vi "load_project.vi"(8 "error in (no error)":errorcluster, 11 "project_file":path) -> (0 "error out":errorcluster, 1 "config":T3, 2 "lv-builder out":refnum<class "lv-builder.lvclass">, 3 "build_spec_info []":T1[](array[typedef]))   [LabVIEW 2015, in "lv-build-interface.lvlib"]
uses:
  lv-build-interface.lvlib
  lv-builder/lv-builder.lvclass
  lv-build/public/_controls/configuration.ctl
  lv-build/public/_controls/build_specification.ctl
  lv-build/public/_controls/build_type.ctl
  lv-build/lv-build.lvlib
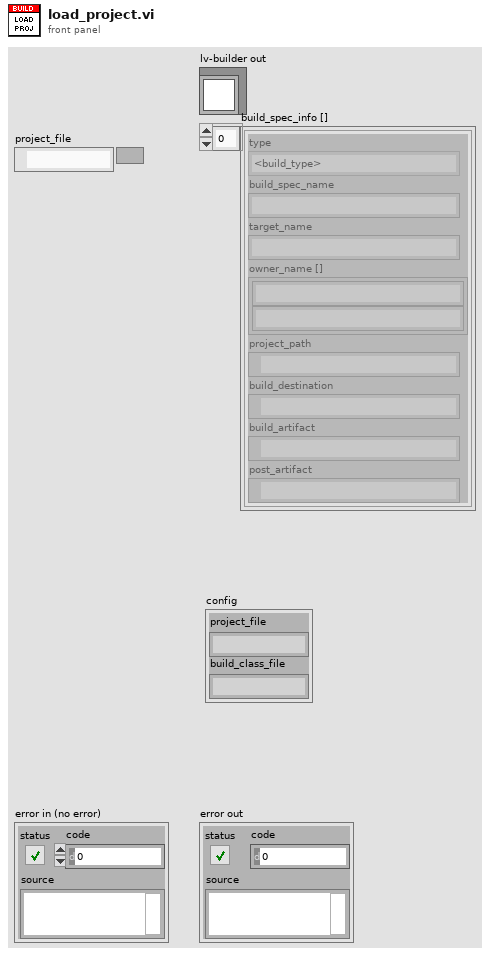
[diagram p1: front panel]
types:
  T1 = typedef "lv-build.lvlib/build_specification.ctl" = cluster{"type":T2, "build_spec_name":string, "target_name":string, "owner_name []":string[], "project_path":path, "build_destination":path, "build_artifact":path, "post_artifact":path}
  T2 = typedef "lv-build.lvlib/build_type.ctl" = enum16{"<build_type>", "application_pc", "application_rt", "installer", "llb", "lvlibp", "zip", "fpga", "<null>"}
  T3 = typedef "lv-build.lvlib/configuration.ctl" = cluster{"project_file":string, "build_class_file":string}
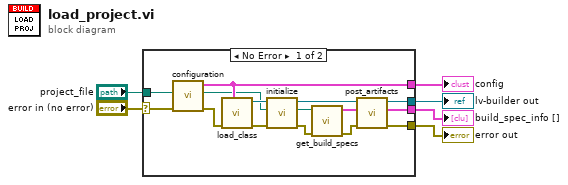
[diagram p0: block diagram]
diagram:
  n1 = case shown="No Error" "error in (no error)" {
    selector: "error in (no error)" -> [w19 w20]
    tunnel: [w10 _] -> w6
    tunnel: [w16 _] -> w4
    tunnel: [w12 w20] -> w3
    tunnel: [w13 _] -> w2
    tunnel: "project_file" -> [w8 _]
    frame No Error {
      n2 = call "configuration.vi"("error in (no error)"=w19, "project_file"=w8) -> ("error out"=w17:errorcluster, "config out"=w16:T3)  [unwired: 8 in]
      n3 = call "load_class.vi"("config in"=w16, "error in (no error)"=w17) -> ("error out"=w18:errorcluster, "lv-builder"=w15:refnum<class "lv-builder.lvclass">)  [unwired: 7 in, 1 out]
      n4 = call-dynamic "initialize.vi"("error in (no error)"=w18, "project_file"=w8, "lv-builder in"=w15) -> ("error out"=w7:errorcluster, "lv-builder out"=w14:refnum<class "lv-builder.lvclass">)  [unwired: 7 in]
      n5 = call "get_build_specs.vi"("error in (no error)"=w7, "project path"=w8) -> ("error out"=w9:errorcluster, "build_spec_info []"=w11:T1[])  [unwired: 8 in]
      n6 = call-dynamic "post_artifacts.vi"("error in (no error)"=w9, "build_spec_info [] in"=w11, "lv-builder in"=w14) -> ("error out"=w12:errorcluster, "build_spec_info [] out"=w10:T1[], "lv-builder out"=w13:refnum<class "lv-builder.lvclass">)  [unwired: 6 in]
    }
    frame Error {
    }
  }
  "lv-builder out" <- w2
  "error out" <- w3
  "config" <- w4
  "build_spec_info []" <- w6
